vi "DEBUG.vi"(6 "Message":string, 8 "error in":errorcluster) -> (0 "error out":errorcluster)   [LabVIEW 2024, in "hse-logger.lvlib"]
doc: "Logs a message and the content of the error-cluster.\nAn error on the \"error in\" terminal is duplicated to the \"error dup\" terminal.\n\nDoes not return logging errors!\n\n____\nHAMPEL SOFTWARE ENGINEERING v2.2.2 (2025-01-16 15:41)"
uses:
  <vilib>/Hampel Software Engineering/HSE Logger/hse-logger.lvlib
  <vilib>/Utility/error.llb/Error Cluster From Error Code.vi
  <vilib>/Hampel Software Engineering/HSE Logger/Logger/Logger.lvclass
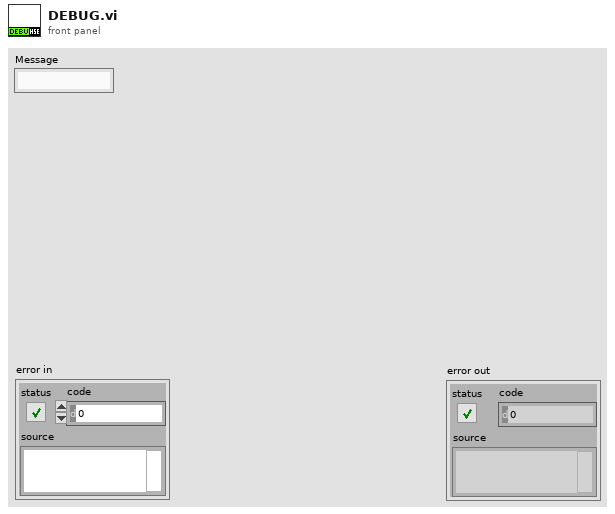
[diagram p1: front panel]
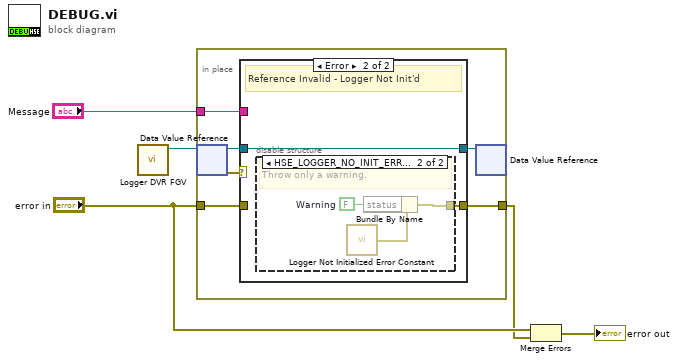
[diagram p0: block diagram]
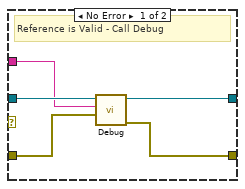
[diagram p2: hidden frame]
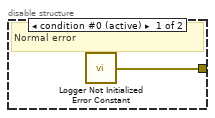
[diagram p3: hidden frame]
diagram:
  n1 = call <vilib>:"Logger DVR FGV.vi"() -> ("Logger DVR"=w2:refnum<data-value>)  [unwired: 10 in, 1 out]
  n2 = in-place {
    in-place-border: "Message" -> [w10]
    in-place-border: [w9] -> w1
    in-place-border: "error in" -> [w6]
    n3 = in-place-dvr #1(w2) -> (w11:refnum<class "Logger.lvclass">, w7:errorcluster)
    n4 = case shown="Error" w7 {
      tunnel: w11 -> [w16 w18]
      tunnel: w10 -> [w15 _]
      tunnel: [w14 w17] -> w9
      tunnel: [w13 w18] -> w8
      tunnel: w6 -> [w12 _]
      frame No Error {
        # "Reference is Valid - Call Debug"
        n5 = call-dynamic "Debug.vi"("Error to Log"=w12, "Message"=w15, "Logger in"=w16) -> ("error out"=w14:errorcluster, "Logger out"=w13:refnum<class "Logger.lvclass">)  [unwired: 7 in]
      }
      frame Error {
        # "Reference Invalid - Logger Not Init'd"
        n6 = disable-structure shown="HSE_LOGGER_NO_INIT_ERROR==True" {
          disable-tunnel: [w19 w21] -> w17
          frame condition #0 (active) {
            # "Normal error"
            n7 = call <vilib>:"Logger Not Initialized Error Constant.vi"() -> ("Logger Not Initialized Error"=w19:errorcluster)
          }
          frame condition #1 {
            w20 = FALSE  # Warning
            # "Throw only a warning."
            n8 = call <vilib>:"Logger Not Initialized Error Constant.vi"() -> ("Logger Not Initialized Error"=w22:errorcluster)
            n9 = Bundle By Name(cluster=w22, "status"=w20) -> (w21:errorcluster)
          }
        }
      }
    }
    n10 = in-place-dvr #1(w8) -> ()  [unwired: 2 out]
  }
  n11 = Merge Errors("error in", w1) -> (→"error out":errorcluster)
